vi "Prosilica Q2D Calibration.vi"() -> ()   [LabVIEW 2012]
uses:
  <vilib>/userdefined/High Color/IMAQdx.ctl
  <vilib>/vision/driver/IMAQdx.llb/IMAQdx Acquisition Mode.ctl
  <vilib>/vision/driver/IMAQdx.llb/IMAQdx Buffer Number Mode.ctl
  <vilib>/Platform/TimedLoop/XDataNode/timing_clust.ctl
  <vilib>/Platform/TimedLoop/XDataNode/nitl_modes.ctl
  <vilib>/Platform/TimedLoop/XDataNode/wakeup.ctl
  <vilib>/Platform/TimedLoop/XDataNode/XDataNode.xnode
  <resource>/objmgr/imaqdx.rc
  <vilib>/vision/driver/NI_Vision_Acquisition_Software.lvlib
  Program Files/Mad City Labs/NanoDrive/Madlib.dll
  <vilib>/Platform/TimedLoop/XDataNode/XDNodeRunTimeDep.lvlib
panel:
  in  "Exposure (us)":dbl(slide)=1407.017543859649 min=100.0 max=15000.0 step=100.0 scale=100.0..15000.0
  in  "Stop VI":bool
  in  "Start Acquisition":bool
  in  "Desired Z Position":dbl=100.0 min=0.0 max=200.0 step=0.01 format="%.4f"
  in  "Desired Y Position":dbl=100.0 min=0.0 max=200.0 step=0.1 format="%.4f"
  out "Current Z Position (um)":dbl format="%.2f"
  out "Current Y Position (um)":dbl format="%.2f"
  in  "Desire X Position":dbl=100.0 min=0.0 max=200.0 step=0.1 format="%.4f"
  out "Current X Position (um)":dbl format="%.2f"
  in  "VISA resource name selected":refnum<visa-resource-name>="COM3"
  in  "Path":path
  out "Frame Number":u32
  out "Frame Rate Out":dbl
  in  "Stop Acquisition":bool
  in  "Number of Frames":u32=18000
  in  "Frame Rate":dbl=5.0
  out "Image":T1(plugin-control)
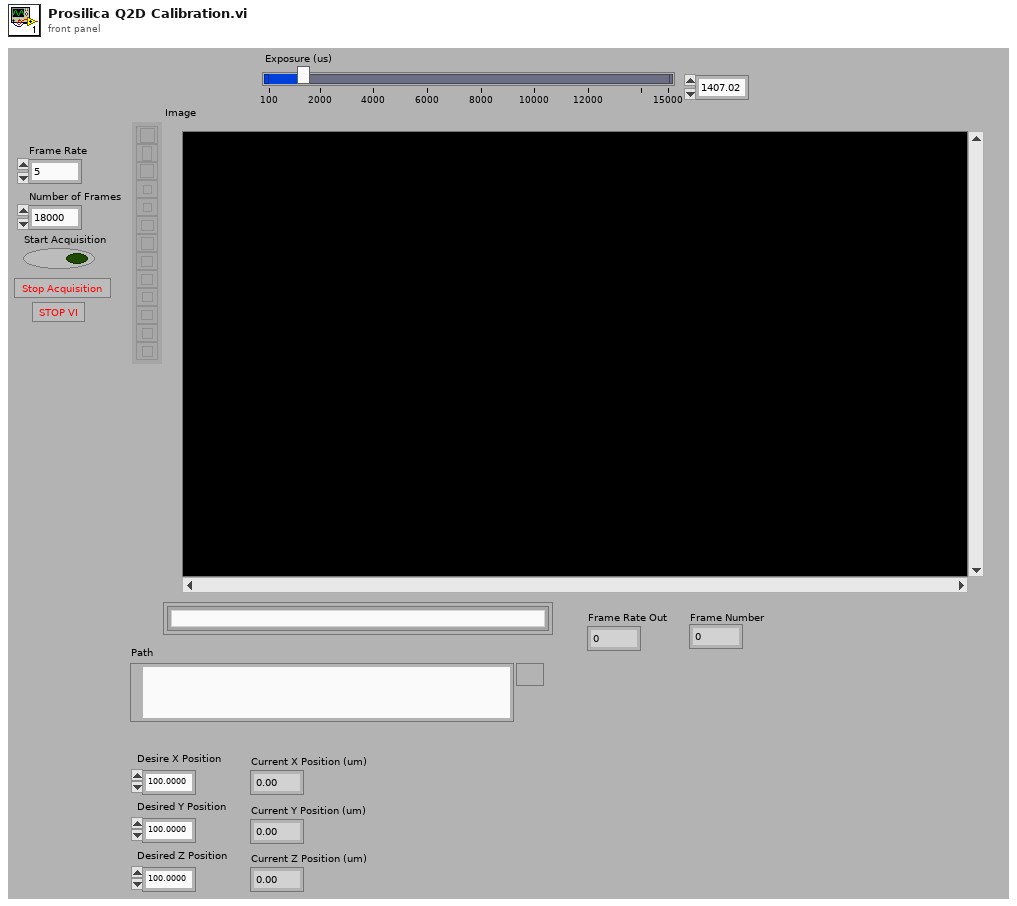
[diagram p1: front panel]
types:
  T1 = typedef "IMAQ Image.ctl" = refnum<image>
  T2 = typedef "IMAQdx.ctl" = refnum<k21>
  T3 = typedef "XDNodeRunTimeDep.lvlib/timing_clust.ctl" = cluster{"Expected End [f-1]":u64, "Actual End [f-1]":u64, "Finished Late? [f-1]":bool, "Expected End [i-1]":u64, "Actual End [i-1]":u64, "Finished Late? [i-1]":bool, "Expected Start [i]":u64, "Actual Start [i]":u64, "Expected Start [f]":u64, "Actual Start [f]":u64, "Source Name":string, "Structure Name":string, "Period":i64, "Deadline":i64, "Offset":i64, "Start":i64, "Priority":i32, "Timeout":i32, "Mode":T4, "Wakeup Reason":T5, "Error":errorcluster, "Source Type":string, "Secondary Source Type":string, "Global End Time":u64, "Global Start Time":u64, "Frame Duration":u64, "Iteration Duration":u64, "Assigned CPU":i32, "I/O Scan Engine Mode":u32}
  T4 = typedef "XDNodeRunTimeDep.lvlib/nitl_modes.ctl" = enum32{"No Change", "Process missed periods, maintain original phase", "Discard missed periods, maintain original phase", "Process missed periods, ignore original phase", "Discard missed periods, ignore original phase"}
  T5 = typedef "XDNodeRunTimeDep.lvlib/wakeup.ctl" = enum32{"Normal", "Aborted", "Asynchronous wakeup", "Timing source error", "Timed loop error", "Timeout"}
  T6 = typedef "NI_Vision_Acquisition_Software.lvlib/IMAQdx Acquisition Mode.ctl" = enum32{"One Shot", "Continuous"}
  T7 = typedef "NI_Vision_Acquisition_Software.lvlib/IMAQdx Buffer Number Mode.ctl" = enum32{"Next", "Last", "Buffer Number"}
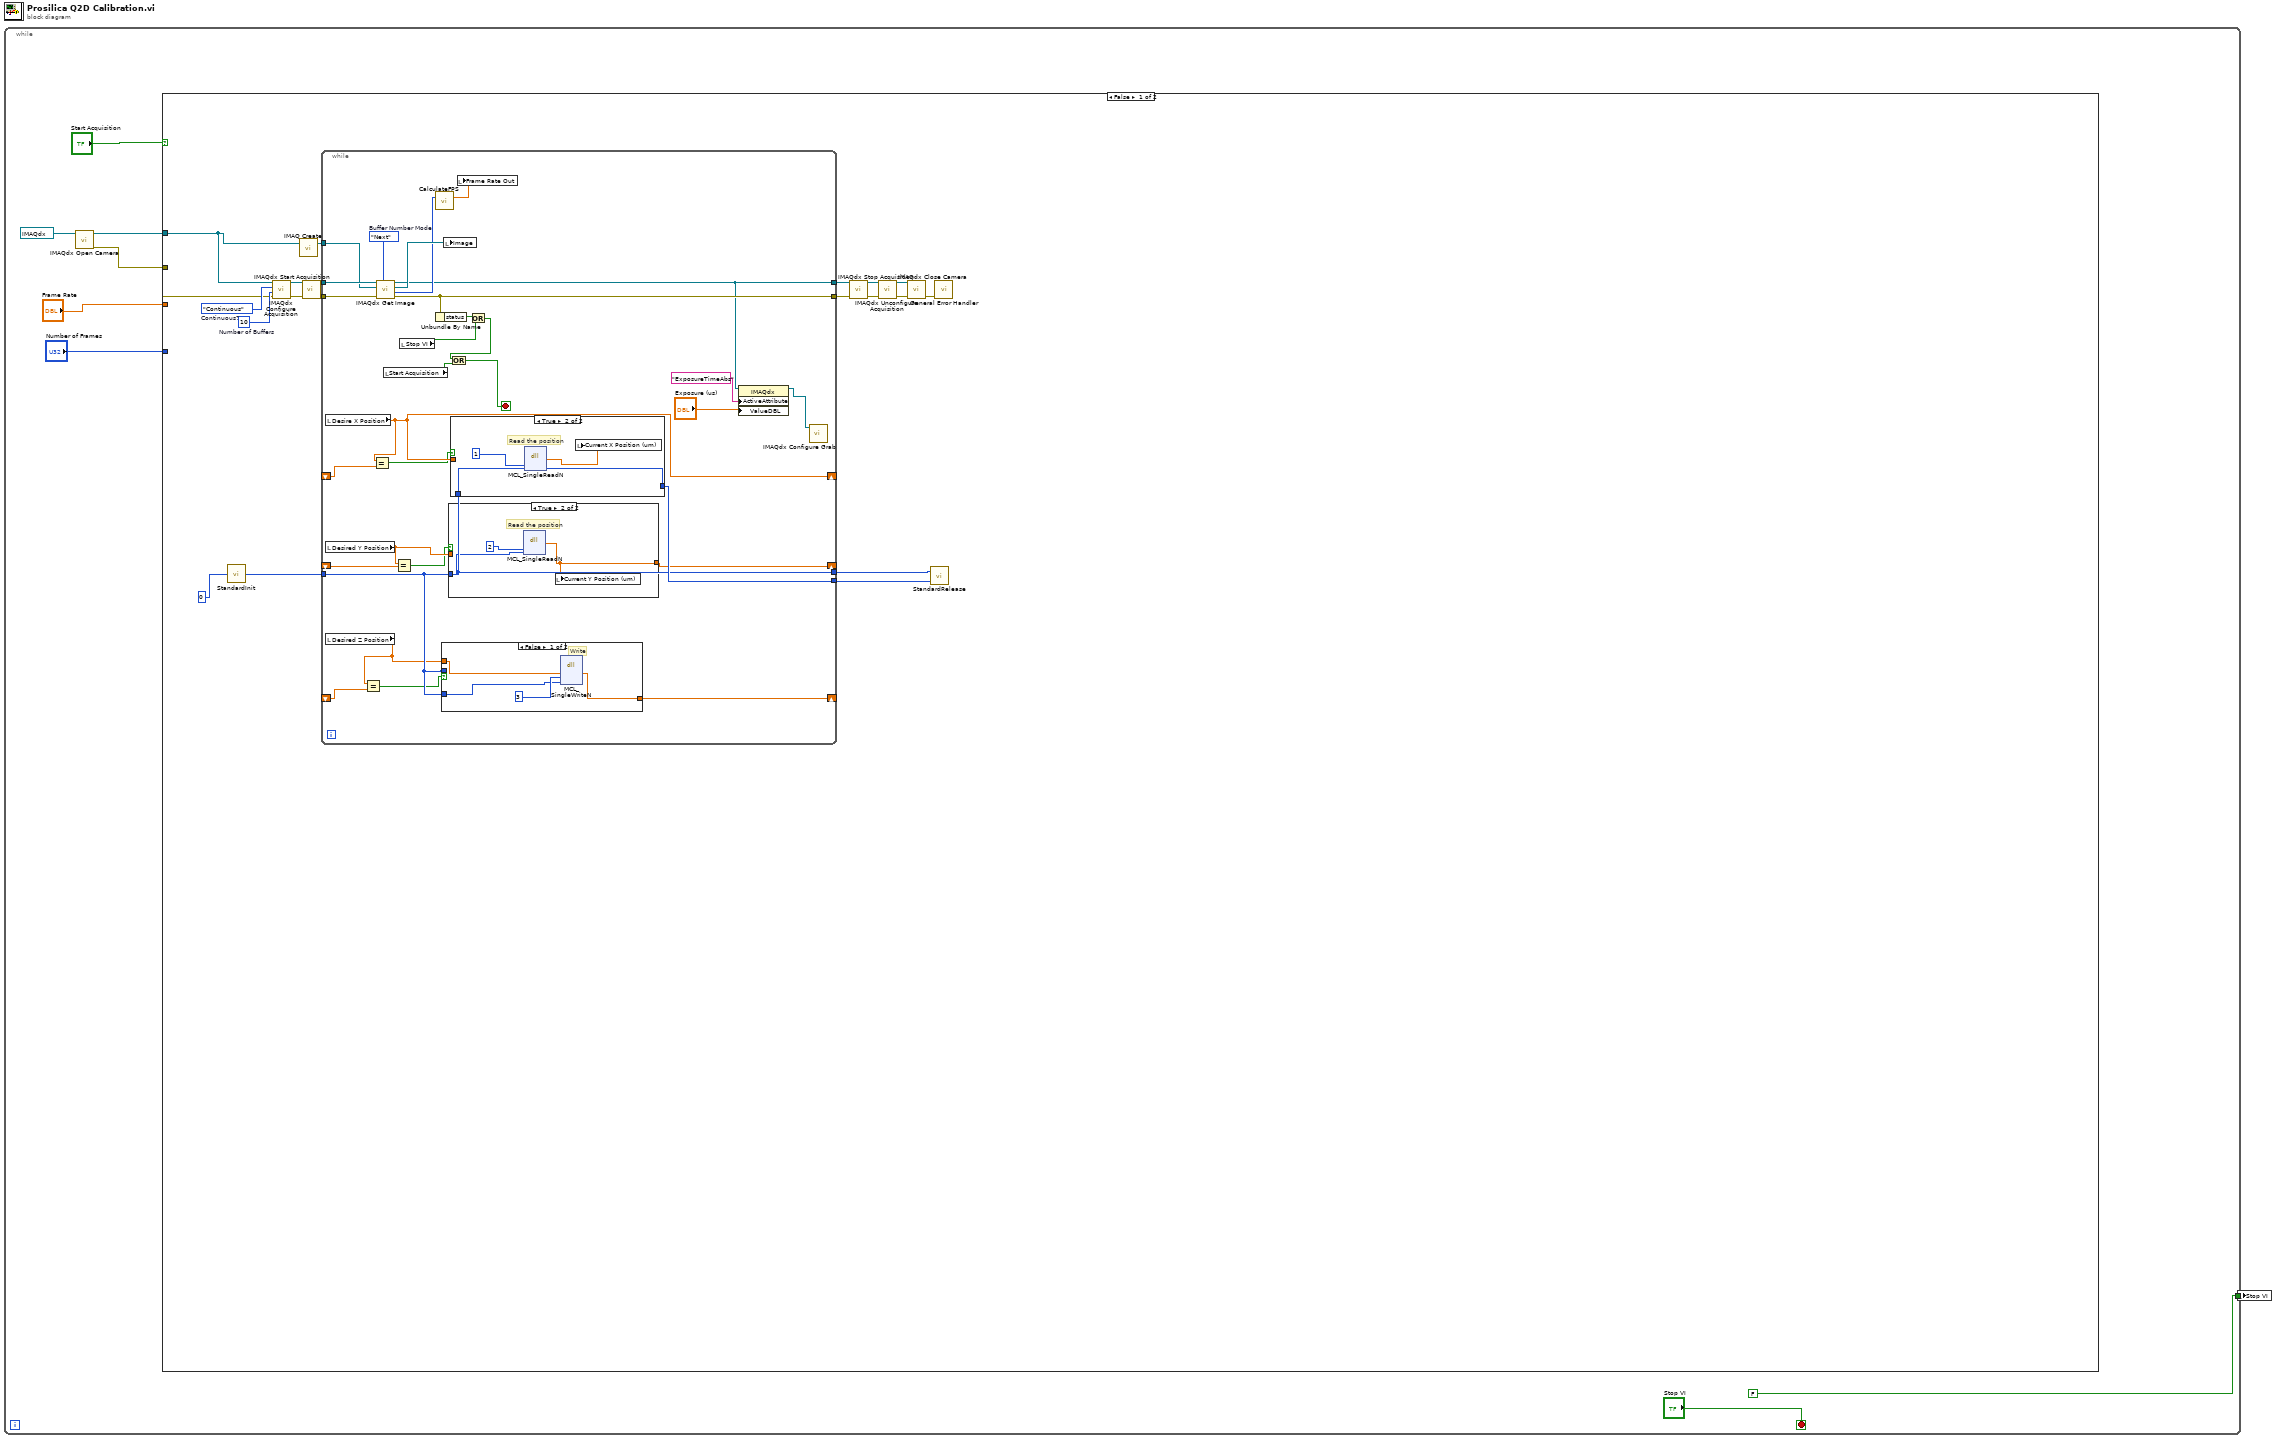
[diagram p0: block diagram]
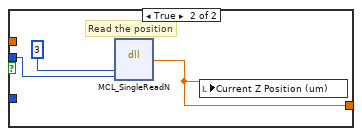
[diagram p2: hidden frame]
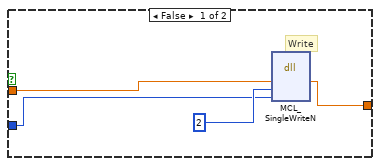
[diagram p3: hidden frame]
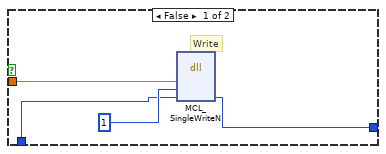
[diagram p4: hidden frame]
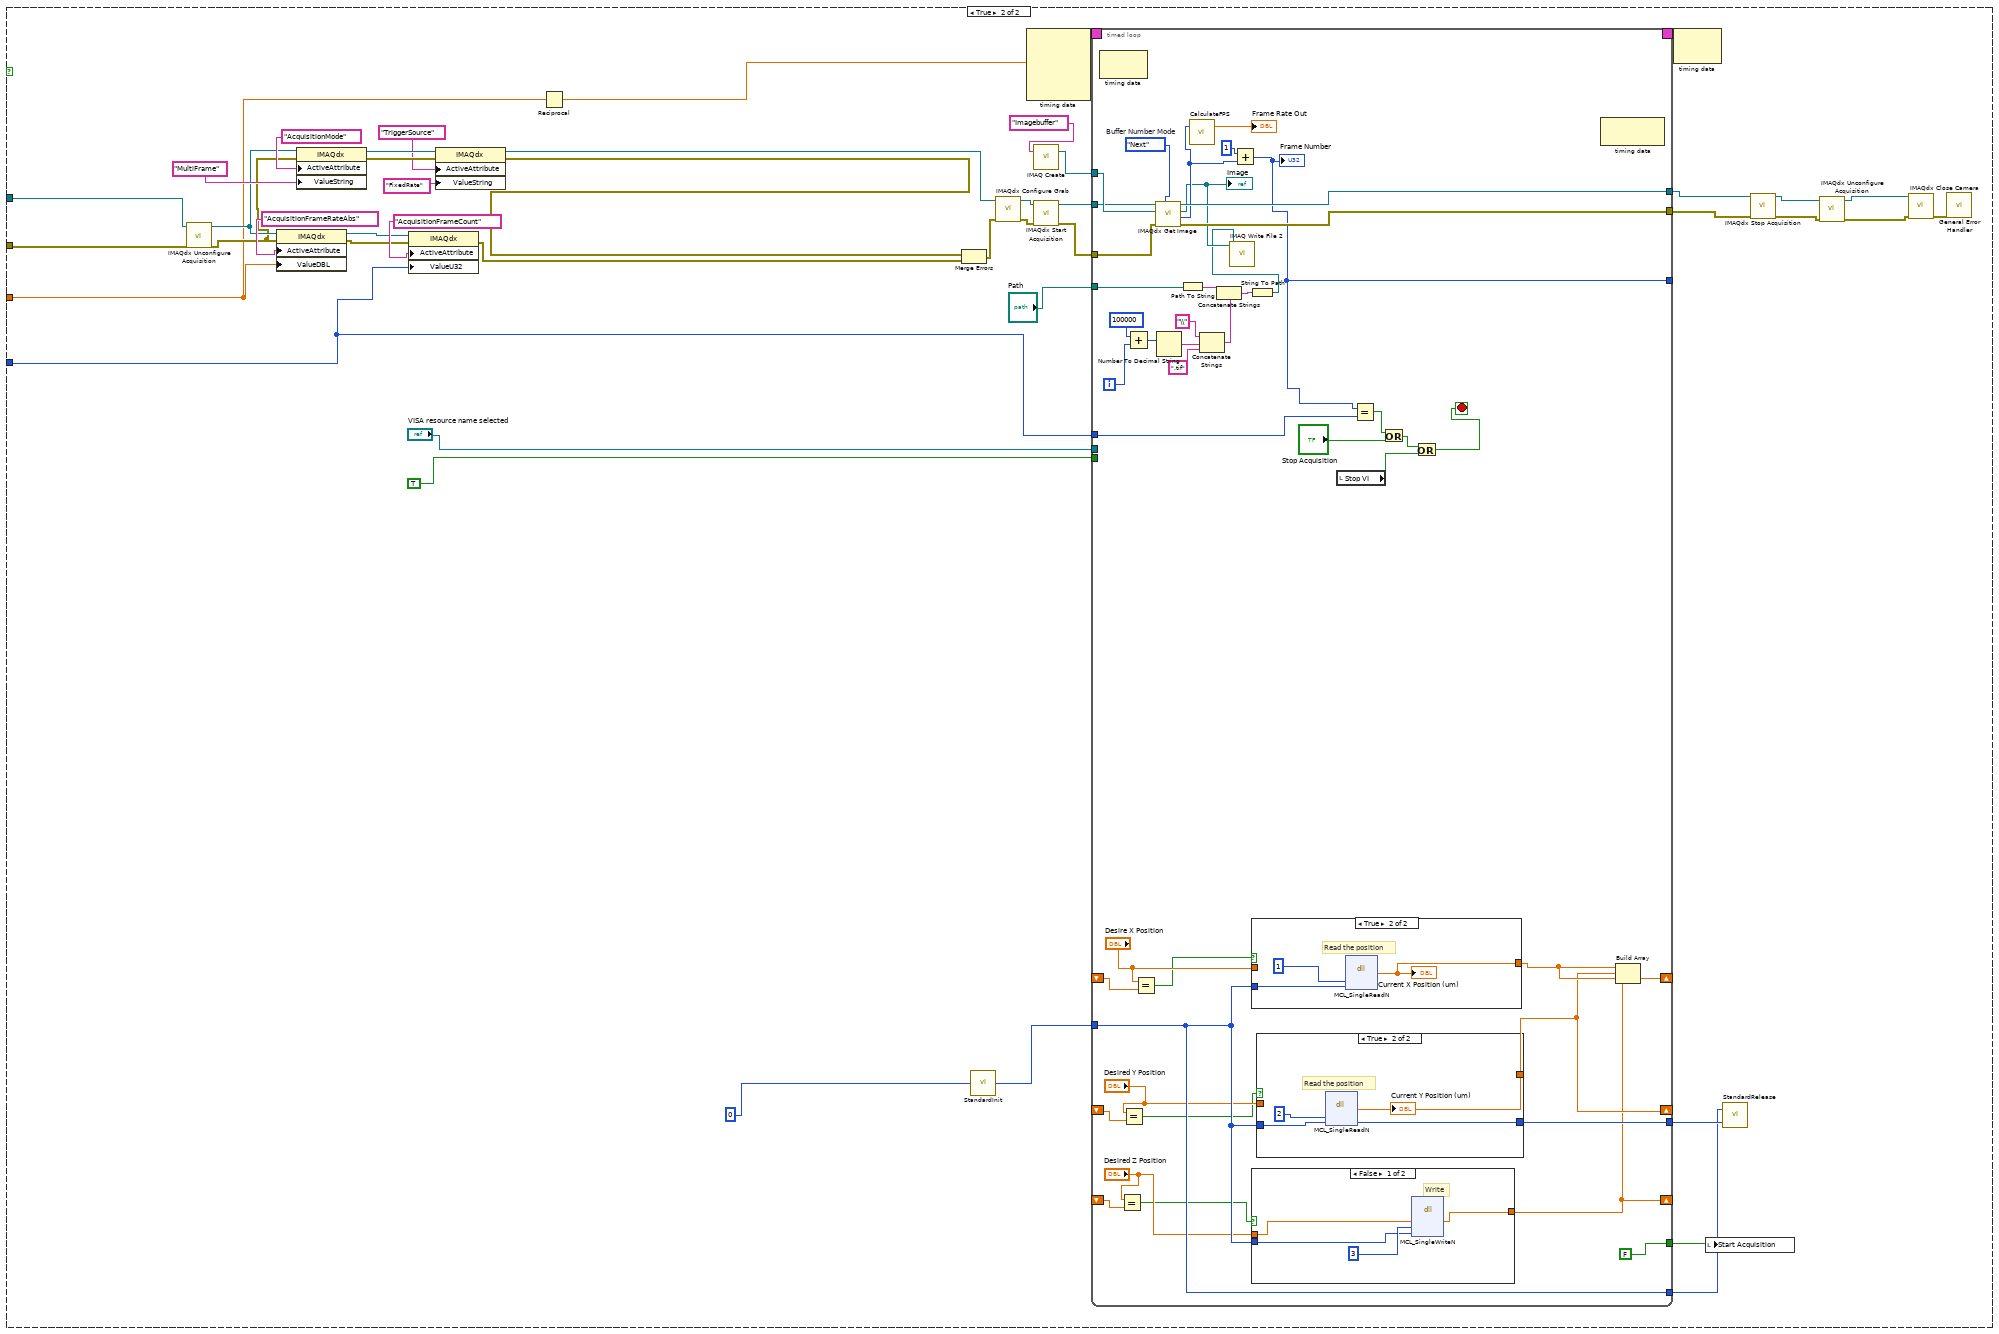
[diagram p5: hidden frame]
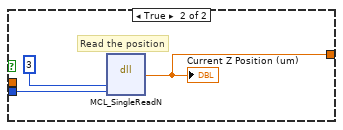
[diagram p6: hidden frame]
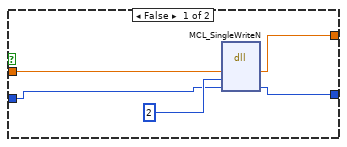
[diagram p7: hidden frame]
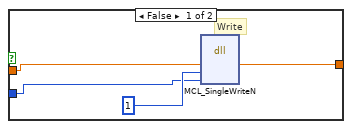
[diagram p8: hidden frame]
diagram:
  n1 = while {
    tunnel: [FALSE] -> w1
    stop <- "Stop VI" stop-if-true
    n2 = call <vilib>:"IMAQdx Open Camera.vi"("Session In"=T2 "cam0") -> ("error out"=w4:errorcluster, "Session Out"=w5:T2)  [unwired: 2 in, 7 out]
    n3 = case shown="False" "Start Acquisition" {
      tunnel: "Frame Rate" -> [_ w83]
      tunnel: "Number of Frames" -> [_ w86]
      tunnel: w5 -> [w20 w99]
      tunnel: w4 -> [w19 w98]
      frame False {
        w26 = IMAQdx_Acquisition_Mode."Continuous"  # Continuous?
        w25 = u32 10  # Number of Buffers
        n4 = call "StandardInit.vi"("Incoming Handle"=0) -> ("Outgoing Handle"=w12:i32)
        n5 = call <vilib>:"IMAQdx Configure Acquisition.vi"("error in"=w19, "Number of Buffers"=w25, "Continuous?"=w26, "Session In"=w20) -> ("error out"=w27:errorcluster, "Session Out"=w28:T2)  [unwired: 6 out]
        n6 = call "IMAQ Create"("Image Name"=w20) -> ("New Image"=w14:T1)  [unwired: 3 in, 2 out]
        n7 = call <vilib>:"IMAQdx Start Acquisition.vi"("error in"=w27, "Session In"=w28) -> ("error out"=w18:errorcluster, "Session Out"=w17:T2)  [unwired: 8 out]
        n8 = while {
          tunnel: w18 -> [w57]
          tunnel: w17 -> [w56]
          tunnel: [w30] -> w16
          tunnel: [w53] -> w15
          tunnel: w14 -> [w52]
          shift-right: [w45] -> _
          shift-left: _ -> [w46]
          tunnel: w12 -> [w40]
          tunnel: [w43] -> w11
          tunnel: [w40] -> w10
          shift-right: [w42] -> _
          shift-left: _ -> [w39]
          shift-right: [w41] -> _
          shift-left: _ -> [w36]
          stop <- w47 stop-if-true
          w58 = IMAQdx_Buffer_Number_Mode."Next"  # Buffer Number Mode
          n9 = local read "Desire X Position"() -> (w45:dbl)
          n10 = local read "Desired Y Position"() -> (w38:dbl)
          n11 = local read "Desired Z Position"() -> (w35:dbl)
          n12 = Equal?(x=w35, y=w36) -> (x = y?=w34:bool)
          n13 = Equal?(x=w45, y=w46) -> (x = y?=w44:bool)
          n14 = call <vilib>:"IMAQdx Get Image.vi"("Buffer Number Mode (Next)"=w58, "error in"=w57, "Image In"=w52, "Session In"=w56) -> ("error out"=w53:errorcluster, "Buffer Number Out"=w51:u32, "Image Out"=w55:T1, "Session Out"=w30:T2)  [unwired: 1 in, 3 out]
          n15 = local read "Start Acquisition"() -> (w49:bool)
          n16 = Equal?(x=w38, y=w39) -> (x = y?=w37:bool)
          n17 = local read "Stop VI"() -> (w50:bool)
          n18 = call "CalculateFPS.vi"("buffer number"=w51) -> ("acquired FPS"=w54:dbl)  [unwired: 2 out]
          n19 = Unbundle By Name(w53) -> ("status"=w59:bool)
          n20 = case shown="False" w34 {
            tunnel: w35 -> [w62 _]
            tunnel: [w61 w64] -> w41
            tunnel: w40 -> [w60 _]
            tunnel: w40 -> [_ w65]
            frame False {
              # "Write"
              n21 = dll-call lib="C:/Program Files/Mad City Labs/NanoDrive/Madlib.dll" fn="MCL_SingleWriteN"("position"=w62, "axis"=u32 3, "handle"=w60) -> ("position"=w61:dbl)  [unwired: 5 in, 3 out]
            }
            frame True {
              # "Read the position"
              n22 = dll-call lib="C:/Program Files/Mad City Labs/NanoDrive/Madlib.dll" fn="MCL_SingleReadN"("axis"=u32 3, "handle"=w65) -> (w64:dbl)  [unwired: 5 in, 2 out]
              n23 = local write "Current Z Position (um)"(w64) -> ()
            }
          }
          n24 = local write "Image"(w55) -> ()
          n25 = case shown="True" w37 {
            tunnel: [w69 w71] -> w42
            tunnel: w38 -> [w68 _]
            tunnel: w40 -> [w67 w72]
            frame False {
              # "Write"
              n26 = dll-call lib="C:/Program Files/Mad City Labs/NanoDrive/Madlib.dll" fn="MCL_SingleWriteN"("position"=w68, "axis"=u32 2, "handle"=w67) -> ("position"=w69:dbl)  [unwired: 5 in, 3 out]
            }
            frame True {
              # "Read the position"
              n27 = dll-call lib="C:/Program Files/Mad City Labs/NanoDrive/Madlib.dll" fn="MCL_SingleReadN"("axis"=u32 2, "handle"=w72) -> ("return type"=w71:dbl)  [unwired: 5 in, 2 out]
              n28 = local write "Current Y Position (um)"(w71) -> ()
            }
          }
          n29 = case shown="True" w44 {
            tunnel: w45 -> [w76 _]
            tunnel: w40 -> [w75 w79]
            tunnel: [w74 w78] -> w43
            frame False {
              # "Write"
              n30 = dll-call lib="C:/Program Files/Mad City Labs/NanoDrive/Madlib.dll" fn="MCL_SingleWriteN"("position"=w76, "axis"=u32 1, "handle"=w75) -> ("handle"=w74:i32)  [unwired: 5 in, 3 out]
            }
            frame True {
              # "Read the position"
              n31 = dll-call lib="C:/Program Files/Mad City Labs/NanoDrive/Madlib.dll" fn="MCL_SingleReadN"("axis"=u32 1, "handle"=w79) -> (w80:dbl, "handle"=w78:i32)  [unwired: 4 in, 2 out]
              n32 = local write "Current X Position (um)"(w80) -> ()
            }
          }
          n33 = local write "Frame Rate Out"(w54) -> ()
          n34 = Or(x=w59, y=w50) -> (x .or. y?=w48:bool)
          n35 = Or(x=w48, y=w49) -> (x .or. y?=w47:bool)
          n36 = property class="IMAQdx"(reference=w30, "ActiveAttribute"="ExposureTimeAbs", "ValueDBL"="Exposure (us)") -> (reference out=w31:T2)  [unwired: 1 in, 1 out]
          n37 = call <vilib>:"IMAQdx Configure Grab.vi"("Session In"=w31) -> ()  [unwired: 9 in, 2 out]
        }
        n38 = call <vilib>:"IMAQdx Stop Acquisition.vi"("error in"=w15, "Session In"=w16) -> ("error out"=w21:errorcluster, "Session Out"=w22:T2)  [unwired: 8 out]
        n39 = call <vilib>:"IMAQdx Unconfigure Acquisition.vi"("error in"=w21, "Session In"=w22) -> ("error out"=w24:errorcluster, "Session Out"=w23:T2)  [unwired: 8 out]
        n40 = call <vilib>:"IMAQdx Close Camera.vi"("error in"=w24, "Session In"=w23) -> ("error out"=w29:errorcluster)  [unwired: 9 out]
        n41 = call "StandardRelease.vi"("Outgoing Handle"=w11, "Incoming Handle"=w10) -> ()  [unwired: 1 out]
        n42 = call <vilib>:"General Error Handler.vi"("error in (no error)"=w29) -> ()  [unwired: 1 in, 14 out]
      }
      frame True {
        n43 = call <vilib>:"IMAQdx Unconfigure Acquisition.vi"("error in"=w98, "Session In"=w99) -> ("error out"=w106:errorcluster, "Session Out"=w109:T2)  [unwired: 8 out]
        n44 = property class="IMAQdx"(reference=w109, error in=w106, "ActiveAttribute"="AcquisitionFrameRateAbs", "ValueDBL"=w83) -> (reference out=w123:T2, error out=w122:errorcluster)
        n45 = property class="IMAQdx"(reference=w109, error in=w106, "ActiveAttribute"="AcquisitionMode", "ValueString"="MultiFrame") -> (reference out=w119:T2, error out=w118:errorcluster)
        n46 = property class="IMAQdx"(reference=w123, error in=w122, "ActiveAttribute"="AcquisitionFrameCount", "ValueU32"=w86) -> (error out=w114:errorcluster)  [unwired: 1 out]
        n47 = property class="IMAQdx"(reference=w119, error in=w118, "ActiveAttribute"="TriggerSource", "ValueString"="FixedRate") -> (reference out=w115:T2, error out=w113:errorcluster)
        n48 = Reciprocal(x=w83) -> (1/x=w82:dbl)
        n49 = Merge Errors(w113, w114) -> (w112:errorcluster)
        n50 = call "StandardInit.vi"("Incoming Handle"=0) -> ("Outgoing Handle"=w104:i32)
        n51 = call <vilib>:"IMAQdx Configure Grab.vi"("error in"=w112, "Session In"=w115) -> ("error out"=w92:errorcluster, "Session Out"=w93:T2)  [unwired: 8 out]
        n52 = node-c288(w82) -> (w85:T3)  [unwired: 3 out]
        n53 = call "IMAQ Create"("Image Name"="Imagebuffer") -> ("New Image"=w111:T1)  [unwired: 3 in, 2 out]
        n54 = call <vilib>:"IMAQdx Start Acquisition.vi"("error in"=w92, "Session In"=w93) -> ("error out"=w91:errorcluster, "Session Out"=w94:T2)  [unwired: 8 out]
        n55 = timed-loop {
          tunnel: w94 -> [w126]
          tunnel: w91 -> [w168]
          tunnel: w111 -> [w167]
          tunnel: [w165] -> w90
          tunnel: [w164] -> w89
          tunnel: "Path" -> [w156]
          tunnel: TRUE -> [_]
          tunnel: "VISA resource name selected" -> [_]
          tunnel: w86 -> [w152]
          tunnel: w104 -> [w149]
          tunnel: [w150] -> w103
          tunnel: [w149] -> w102
          tunnel: [FALSE] -> w95
          shift-right: [w143] -> _
          shift-left: _ -> [w142]
          shift-right: [w139] -> _
          shift-left: _ -> [w138]
          shift-right: [w135] -> _
          shift-left: _ -> [w134]
          timing: w85 -> [_]
          timing-out: [_] -> w84
          tunnel: [w127] -> _
          i -> [w131]
          stop <- w146 stop-if-true
          w144 = IMAQdx_Buffer_Number_Mode."Next"  # Buffer Number Mode
          n56 = node-c288() -> ()  [unwired: 2 out]
          n57 = Equal?(x="Desired Z Position", y=w134) -> (x = y?=w132:bool)
          n58 = Equal?(x="Desired Y Position", y=w138) -> (x = y?=w136:bool)
          n59 = Add(x=100000, y=w131) -> (x+y=w129:i32)
          n60 = Equal?(x="Desire X Position", y=w142) -> (x = y?=w140:bool)
          n61 = call <vilib>:"IMAQdx Get Image.vi"("Buffer Number Mode (Next)"=w144, "error in"=w168, "Image In"=w167, "Session In"=w126) -> ("error out"=w164:errorcluster, "Buffer Number Out"=w163:u32, "Image Out"=w162:T1, "Session Out"=w165:T2)  [unwired: 1 in, 3 out]
          "Image" <- w162
          n62 = Number To Decimal String(number=w129) -> (decimal integer string=w159:string)  [unwired: 1 out]
          n63 = Path To String(path=w156) -> (string=w161:string)
          n64 = call "CalculateFPS.vi"("buffer number"=w163) -> ("acquired FPS"=→"Frame Rate Out":dbl)  [unwired: 2 out]
          n65 = Concatenate Strings("\\" ("string"), w159, ".tif") -> (w157:string)
          n66 = Concatenate Strings(w161, w157) -> (w160:string)
          n67 = Add(x=1, y=w163) -> (x+y=w127:u32)
          "Frame Number" <- w127
          n68 = String To Path(string=w160) -> (path=w155:path)
          n69 = call-poly "IMAQ Write File 2"("File Path"=w155, "Image"=w162) -> ()  [unwired: 3 in, 7 out]
          n70 = case shown="True" w140 {
            tunnel: w149 -> [w188 w193]
            tunnel: [w187 w192] -> w143
            tunnel: "Desire X Position" -> [w189 _]
            frame False {
              # "Write"
              n71 = dll-call lib="C:/Program Files/Mad City Labs/NanoDrive/Madlib.dll" fn="MCL_SingleWriteN"("position"=w189, "axis"=u32 1, "handle"=w188) -> ("position"=w187:dbl)  [unwired: 5 in, 3 out]
            }
            frame True {
              # "Read the position"
              n72 = dll-call lib="C:/Program Files/Mad City Labs/NanoDrive/Madlib.dll" fn="MCL_SingleReadN"("axis"=u32 1, "handle"=w193) -> (w192:dbl)  [unwired: 5 in, 2 out]
              "Current X Position (um)" <- w192
            }
          }
          n73 = case shown="False" w132 {
            tunnel: w149 -> [w171 w177]
            tunnel: [w172 w176] -> w135
            tunnel: "Desired Z Position" -> [w173 _]
            frame False {
              # "Write"
              n74 = dll-call lib="C:/Program Files/Mad City Labs/NanoDrive/Madlib.dll" fn="MCL_SingleWriteN"("position"=w173, "axis"=u32 3, "handle"=w171) -> ("position"=w172:dbl)  [unwired: 5 in, 3 out]
            }
            frame True {
              # "Read the position"
              n75 = dll-call lib="C:/Program Files/Mad City Labs/NanoDrive/Madlib.dll" fn="MCL_SingleReadN"("axis"=u32 3, "handle"=w177) -> (w176:dbl)  [unwired: 5 in, 2 out]
              "Current Z Position (um)" <- w176
            }
          }
          n76 = case shown="True" w136 {
            tunnel: [w178 w186] -> w150
            tunnel: w149 -> [w180 w185]
            tunnel: [w179 w184] -> w139
            tunnel: "Desired Y Position" -> [w181 _]
            frame False {
              n77 = dll-call lib="C:/Program Files/Mad City Labs/NanoDrive/Madlib.dll" fn="MCL_SingleWriteN"("position"=w181, "axis"=u32 2, "handle"=w180) -> ("position"=w179:dbl, "handle"=w178:i32)  [unwired: 4 in, 3 out]
            }
            frame True {
              # "Read the position"
              n78 = dll-call lib="C:/Program Files/Mad City Labs/NanoDrive/Madlib.dll" fn="MCL_SingleReadN"("axis"=u32 2, "handle"=w185) -> (w184:dbl, "handle"=w186:i32)  [unwired: 4 in, 2 out]
              "Current Y Position (um)" <- w184
            }
          }
          n79 = local read "Stop VI"() -> (w147:bool)
          n80 = Equal?(x=w127, y=w152) -> (x = y?=w151:bool)
          n81 = Or(x=w151, y="Stop Acquisition") -> (x .or. y?=w148:bool)
          n82 = Or(x=w148, y=w147) -> (x .or. y?=w146:bool)
          n83 = node-c288() -> ()  [unwired: 2 out]
          n84 = Build Array(w143, w139, w135) -> ()  [unwired: 1 out]
        }
        n85 = node-c288(w84) -> ()  [unwired: 1 out]
        n86 = local write "Start Acquisition"(w95) -> ()
        n87 = call "StandardRelease.vi"("Outgoing Handle"=w103, "Incoming Handle"=w102) -> ()  [unwired: 1 out]
        n88 = call <vilib>:"IMAQdx Stop Acquisition.vi"("error in"=w89, "Session In"=w90) -> ("error out"=w87:errorcluster, "Session Out"=w88:T2)  [unwired: 8 out]
        n89 = call <vilib>:"IMAQdx Unconfigure Acquisition.vi"("error in"=w87, "Session In"=w88) -> ("error out"=w96:errorcluster, "Session Out"=w97:T2)  [unwired: 8 out]
        n90 = call <vilib>:"IMAQdx Close Camera.vi"("error in"=w96, "Session In"=w97) -> ("error out"=w108:errorcluster)  [unwired: 9 out]
        n91 = call <vilib>:"General Error Handler.vi"("error in (no error)"=w108) -> ()  [unwired: 1 in, 14 out]
      }
    }
  }
  n92 = local write "Stop VI"(w1) -> ()
